vi "LinearConvertionInverse.vi"(0 "Input":dbl, 1 "Calib factors":T1={"a"=1.0, "b"=0.0}) -> (2 "Output":dbl)   [LabVIEW 2012]
uses:
  LinearFactors.ctl
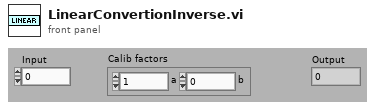
[diagram p1: front panel]
types:
  T1 = typedef "LinearFactors.ctl" = cluster{"a":dbl, "b":dbl}
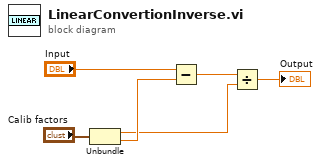
[diagram p0: block diagram]
diagram:
  n1 = Unbundle("Calib factors") -> ("a"=w1:dbl, "b"=w2:dbl)
  n2 = Subtract(x="Input", y=w2) -> (x-y=w4:dbl)
  n3 = Divide(x=w4, y=w1) -> (x/y=→"Output":dbl)
